vi "Generate Error Cluster.vi"(8 "error in (no error)":errorcluster, 10 "Additional Info":string, 11 "Error":T1) -> (0 "error out":errorcluster)   [LabVIEW 2015]
uses:
  Error Code.ctl
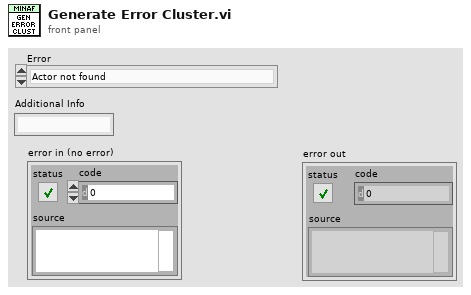
[diagram p1: front panel]
types:
  T1 = typedef "Error Code.ctl" = enum16{"Actor not found", "Wait for reply timed out", "Framework Error", "Actor not OK", "Error Starting Measurement"}
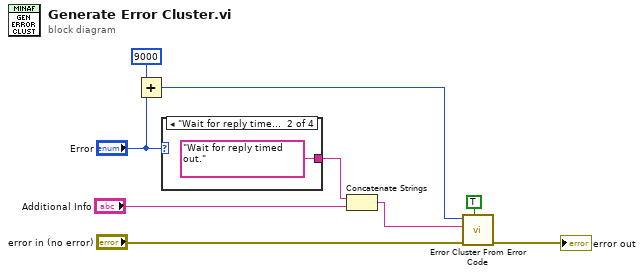
[diagram p0: block diagram]
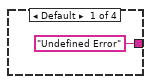
[diagram p2: hidden frame]
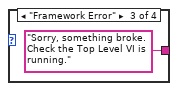
[diagram p3: hidden frame]
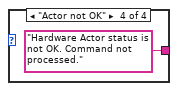
[diagram p4: hidden frame]
diagram:
  n1 = Add(x=9000, y="Error") -> (x+y=w8:i32)
  n2 = case shown="\"Wait for reply timed out\"" "Error" {
    tunnel: ["Undefined Error" "Wait for reply timed out." "Sorry, something broke. Check the Top Level VI is running." "Hardware Actor status is not OK. Command not processed."] -> w1
    frame Default {
    }
    frame "Wait for reply timed out" {
    }
    frame "Framework Error" {
    }
    frame "Actor not OK" {
    }
  }
  n3 = Concatenate Strings(w1, "Additional Info") -> (w2:string)
  n4 = call <vilib>:"Error Cluster From Error Code.vi"("show call chain? (False)"=TRUE, "error in (no error)"="error in (no error)", "error message (\"\")"=w2, "error code (0)"=w8) -> ("error out"=→"error out":errorcluster)  [unwired: 5 in]
